vi "Read FXPIL.vi"(8 "error in (no error)":errorcluster, 11 "Channel_FXP in":refnum<class "Channel_FXP.lvclass">) -> (0 "error out":errorcluster, 2 "FXPIL":i32, 3 "Channel_FXP out":refnum<class "Channel_FXP.lvclass">)   [LabVIEW 2013, in "Channel_FXP.lvclass"]
uses:
  Channel_FXP.lvclass
  Channel_FXP.lvclass/Channel_FXP.ctl
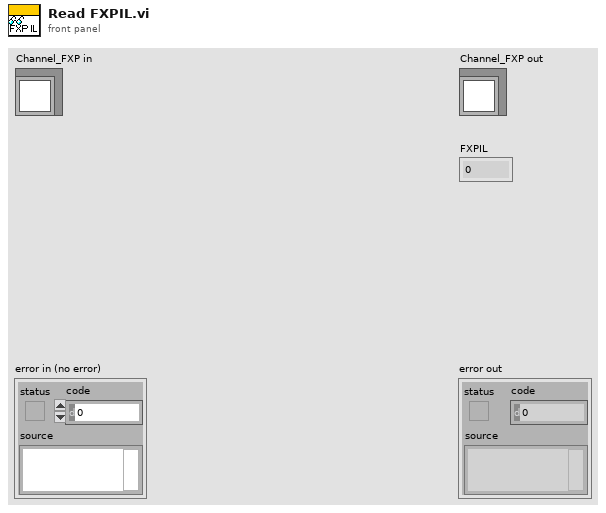
[diagram p1: front panel]
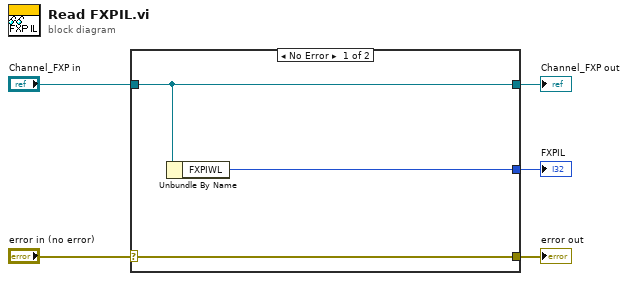
[diagram p0: block diagram]
diagram:
  n1 = case shown="No Error" "error in (no error)" {
    selector: "error in (no error)" -> [w8 w9]
    tunnel: [w8 w9] -> w4
    tunnel: [w7 w10] -> w2
    tunnel: "Channel_FXP in" -> [w7 w10]
    tunnel: [w6 _] -> w1
    frame No Error {
      n2 = Unbundle By Name(w7) -> ("FXPIWL"=w6:i32)
    }
    frame Error {
    }
  }
  "error out" <- w4
  "Channel_FXP out" <- w2
  "FXPIL" <- w1
